vi "Clamp MAX_Setting_UI.vi"(6 "Analysis_Setting IN":T2={"PreProcess"=enum."*Algorithm*", "Parameter"=""}, 8 "error in (no error)":errorcluster, 9 "ProjectName":string, 10 "ROI List IN":refnum<vi>, 11 "Vision_Image":T10(plugin-control)) -> (0 "error out":errorcluster, 1 "Cancel?":bool, 3 "Analysis_Setting":T2={"PreProcess"=enum."*Algorithm*", "Parameter"=""})   [LabVIEW 2019]
uses:
  <vilib>/userdefined/High Color/IMAQdx.ctl
  <vilib>/vision/NI_Vision_Development_Module.lvlib
  Controls/_UI Command Cluster/Clamp MAX_UI Command Cluster.ctl
  Controls/Clamp MAX/Analysis_Clamp MAX_Parameter.ctl
  Controls/Analysis_Type.ctl
  Controls/Analysis_Setting.ctl
  Controls/V_Analysis_Type.ctl
  Ctrl/VisionProcessName.ctl
panel:
  in  "Snap?":bool
  in  "ROI":T1
  in  "Overlay Settings":T4={"Show Search Area"=TRUE, "Show Curves"=TRUE, "Show Clamp Locations"=TRUE, "Show Result"=TRUE, "Search Area Color"=6618880, "Curves Color"=16777224, "Clamp Locations Color"=16776960, "Result Color"=16711680, "Overlay Group Name"=""}
  out "Numeric":i32
  in  "Done":bool
  in  "Clamp MAX_UI Command":T5(ring)
  in  "Cancel":bool
  in  "Clamp MAXTab":T6(tab)
  in  "Clamp Settings":T7={"Angle Range (+/-)"=100.0, "Edge Polarity"={"Start"=0, "End"=0}} {"Edge Polarity"."End" items=["Any", "Rising", "Falling"]; "Edge Polarity"."Start" items=["Any", "Rising", "Falling"]}
  in  "Curve Extraction Settings":T8={"Extraction Mode"=enum."Normal", "Edge Threshold"=40, "Edge Filter Size"=enum."Normal", "Min Length"=15, "Row Search Step Size"=10, "Col Search Step Size"=10, "Max Endpoint Gap"=5, "Closed"=FALSE, "Subpixel"=FALSE} {"Max Endpoint Gap" min=0; "Col Search Step Size" min=1 max=255 step=1; "Row Search Step Size" min=1 max=255 step=1; "Min Length" min=0; "Edge Threshold" min=1 max=350 step=1}
  out "Clamp MAX Results":T9 {"Angle (Relative)" format="%.3f"; "Angle (Absolute)" format="%.3f"; "Distance (Real World)" format="%.3f"; "Distance (Pixels)" format="%.3f"}
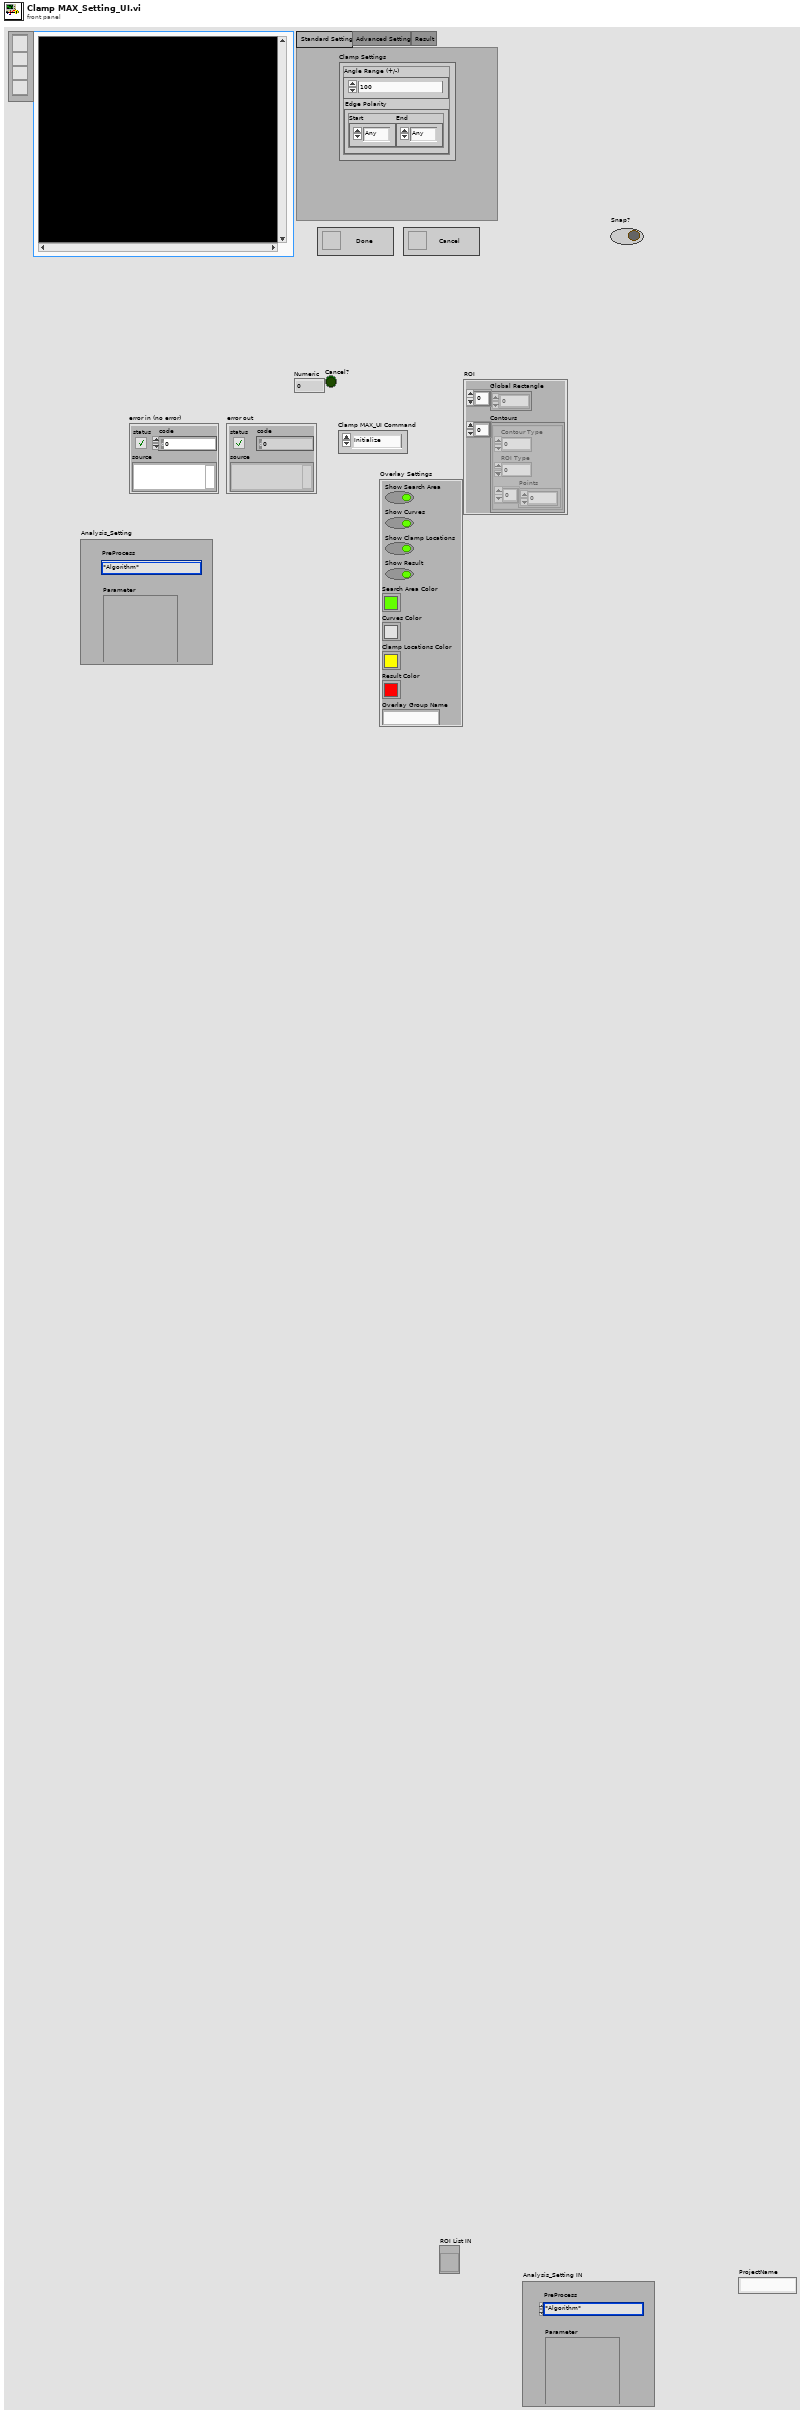
[diagram p1: front panel]
types:
  T1 = cluster{"Global Rectangle":i32[], "Contours":cluster{"Contour Type":u32, "ROI Type":u32, "Points":i32[]}[]}
  T2 = typedef "Analysis_Setting.ctl" = cluster{"PreProcess":T3, "Parameter":string}
  T3 = typedef "VisionProcessName.ctl" = enum16{"*CamParameter*", "CamAttributes", "*Preprocess*", "CG_Brightness", "C_Plane Extraction", "C_Threshold", "G_Lookup Table", "G_Threshold", "B_Image Inversion", "*Algorithm*", "CG_Histogram", "C_Color Matching", "C_Color Pattern Matching", "G_PatternMatch", "CG_Find Straight Edge", "CG_Adv. Find Straight Edge", "CG_Find Circular Edge", "G_Max Clamp", "G_Clamp (Rake)", "G_Pattern Matching"}
  T4 = cluster{"Show Search Area":bool, "Show Curves":bool, "Show Clamp Locations":bool, "Show Result":bool, "Search Area Color":u32, "Curves Color":u32, "Clamp Locations Color":u32, "Result Color":u32, "Overlay Group Name":string}
  T5 = enum16{"Initialize", "Done", "Run Algorithm", "Cancel"}
  T6 = enum32{"Standard Setting", "Advanced Setting", "Result"}
  T7 = cluster{"Angle Range (+/-)":dbl, "Edge Polarity":cluster{"Start":u32, "End":u32}}
  T8 = cluster{"Extraction Mode":enum16{"Normal", "Uniform Regions"}, "Edge Threshold":i32, "Edge Filter Size":enum16{"Fine", "Normal", "Contour Tracing"}, "Min Length":i32, "Row Search Step Size":i32, "Col Search Step Size":i32, "Max Endpoint Gap":i32, "Closed":bool, "Subpixel":bool}
  T9 = cluster{"Distance (Pixels)":dbl, "Distance (Real World)":dbl, "Angle (Absolute)":dbl, "Angle (Relative)":dbl}
  T10 = typedef "IMAQ Image.ctl" = refnum<image>
  T11 = typedef "Clamp MAX_UI Command Cluster.ctl" = cluster{"Clamp MAX_UI Command":enum16{"Initialize", "Done", "Run Algorithm", "Cancel"}, "Overlay Settings":cluster{"Show Search Area":bool, "Show Curves":bool, "Show Clamp Locations":bool, "Show Result":bool, "Search Area Color":u32, "Curves Color":u32, "Clamp Locations Color":u32, "Result Color":u32, "Overlay Group Name":string}, "Curve Extraction Settings":cluster{"Extraction Mode":u32, "Edge Threshold":i32, "Edge Filter Size":u32, "Min Length":i32, "Row Search Step Size":i32, "Col Search Step Size":i32, "Max Endpoint Gap":i32, "Closed":bool, "Subpixel":bool}, "Clamp Settings":cluster{"Angle Range (+/-)":dbl, "Edge Polarity":cluster{"Start":u32, "End":u32}}, "Snap Simulation Mouse Down":bool, "ROI":cluster{"Global Rectangle":i32[], "Contours":cluster{"Contour Type":u32, "ROI Type":u32, "Points":i32[]}[]}}
  T12 = typedef "IMAQ Line" = cluster{"Start X":i32, "Start Y":i32, "End X":i32, "End Y":i32}
  T13 = typedef "IMAQdx.ctl" = refnum<k21>
  T14 = cluster{"Contour Type":u32, "ROI Type":u32, "Points":i32[]}
  T15 = cluster{"Extraction Mode":u32, "Edge Threshold":i32, "Edge Filter Size":u32, "Min Length":i32, "Row Search Step Size":i32, "Col Search Step Size":i32, "Max Endpoint Gap":i32, "Closed":bool, "Subpixel":bool}
  T16 = typedef "Image Type" = u32
  T17 = typedef "Analysis_Clamp MAX_Parameter.ctl" = cluster{"Overlay Settings":cluster{"Show Search Area":bool, "Show Curves":bool, "Show Clamp Locations":bool, "Show Result":bool, "Search Area Color":u32, "Curves Color":u32, "Clamp Locations Color":u32, "Result Color":u32, "Overlay Group Name":string}, "Curve Extraction Settings":cluster{"Extraction Mode":u32, "Edge Threshold":i32, "Edge Filter Size":u32, "Min Length":i32, "Row Search Step Size":i32, "Col Search Step Size":i32, "Max Endpoint Gap":i32, "Closed":bool, "Subpixel":bool}, "Clamp Settings":cluster{"Angle Range (+/-)":dbl, "Edge Polarity":cluster{"Start":u32, "End":u32}}, "ROI":cluster{"Global Rectangle":i32[], "Contours":cluster{"Contour Type":u32, "ROI Type":u32, "Points":i32[]}[]}}
  T18 = typedef "Analysis_Type.ctl" = u16
  T19 = typedef "Analysis_Setting.ctl" = cluster{"PreProcess":T20, "Parameter":string}
  T20 = typedef "V_Analysis_Type.ctl" = enum16{"None", "C_Color Pattern Matching", "G_PatternMatching", "G_ShapeDectect", "G_GeometricMatch", "B_Area Check"}
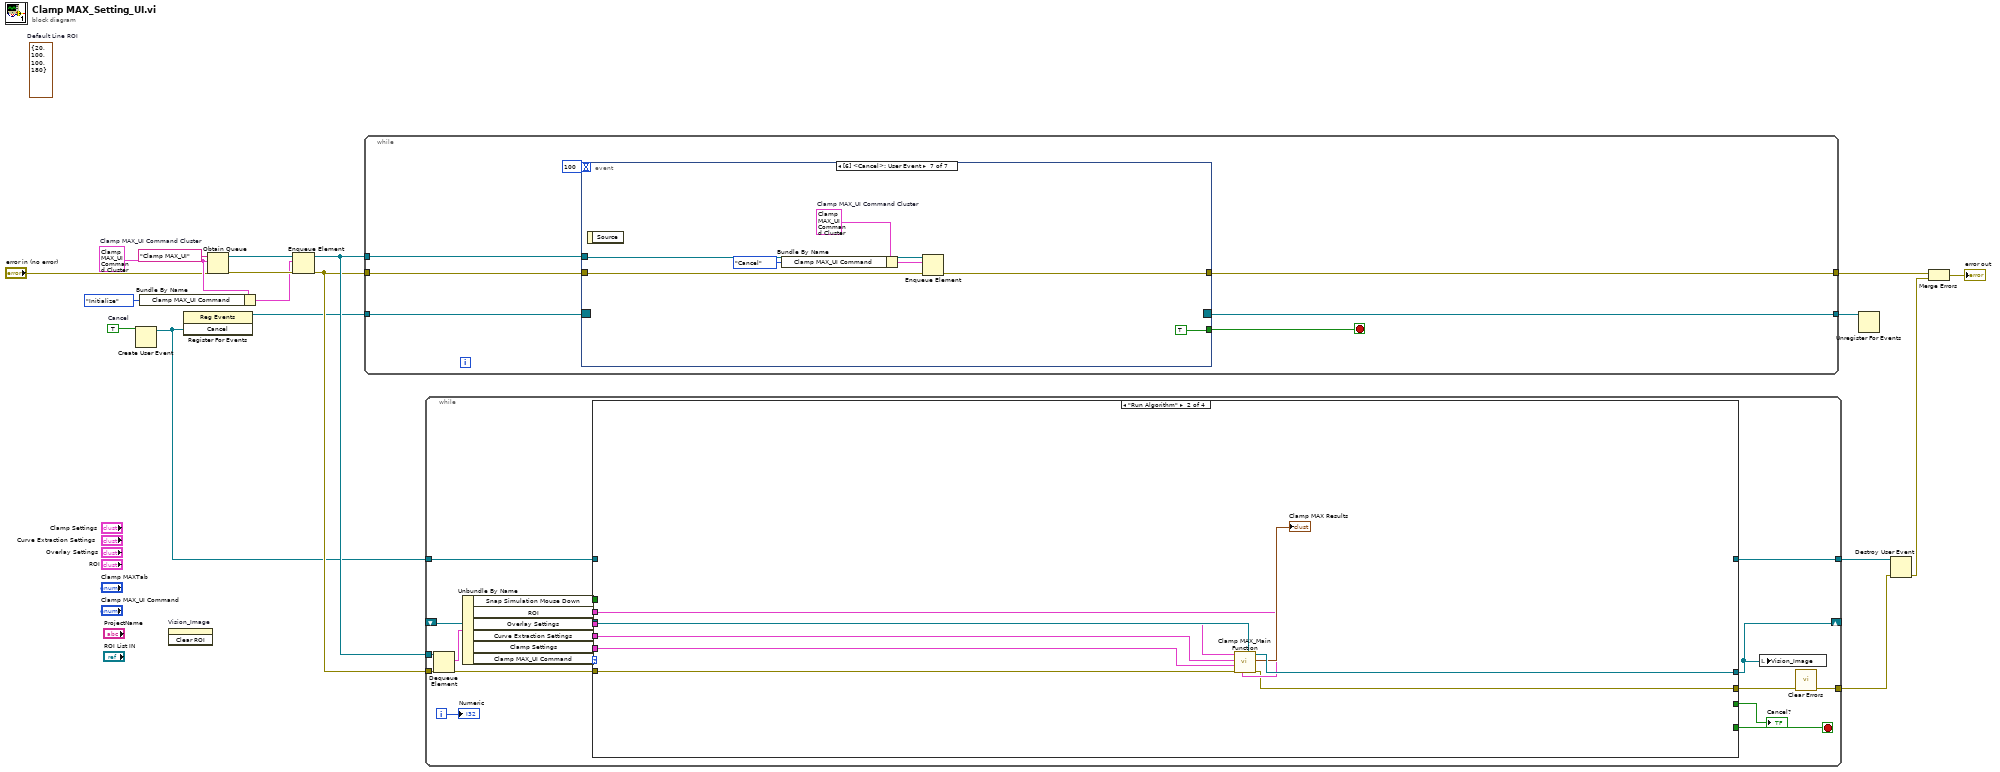
[diagram p0: block diagram]
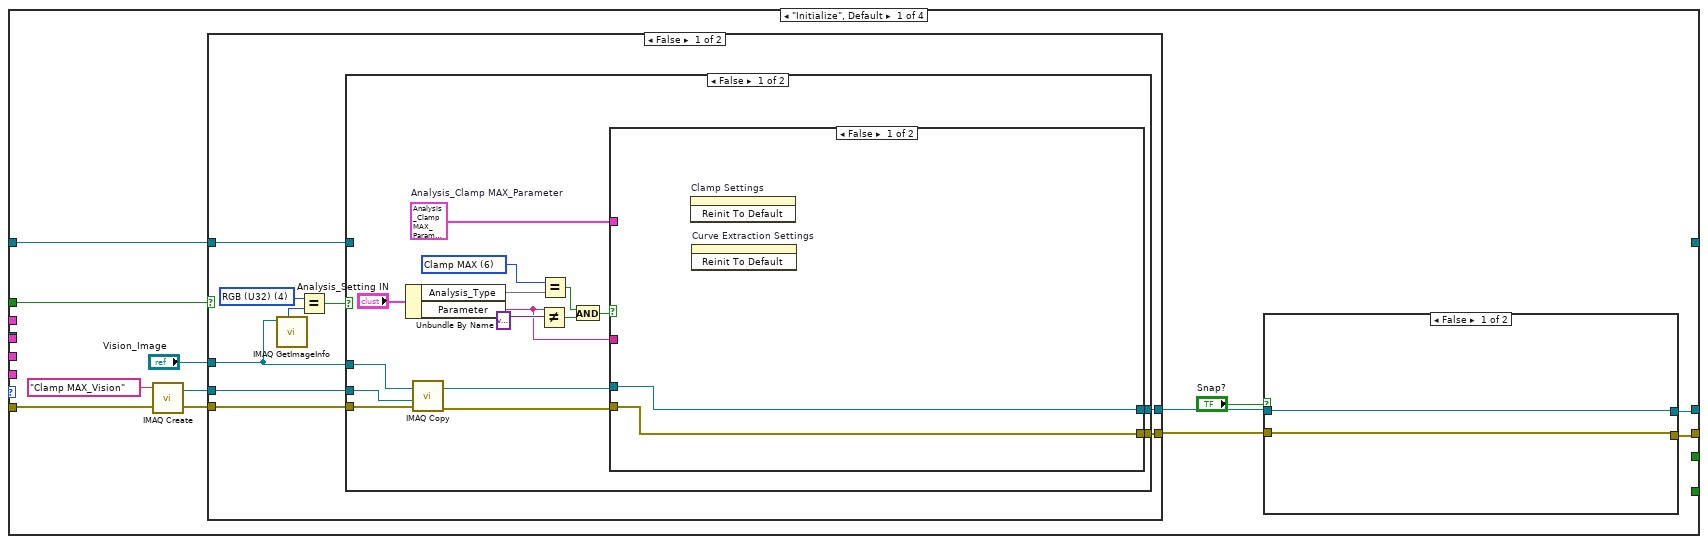
[diagram p2: hidden frame]
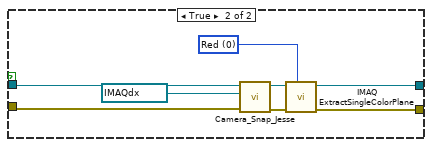
[diagram p3: hidden frame]
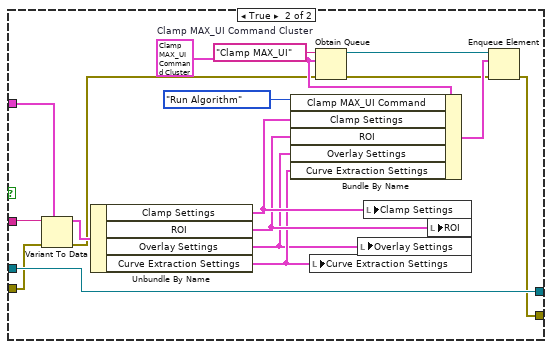
[diagram p4: hidden frame]
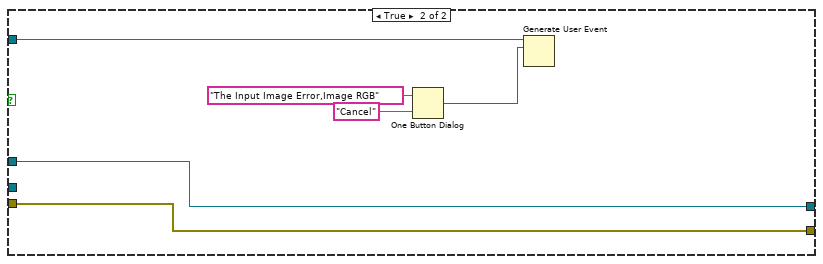
[diagram p5: hidden frame]
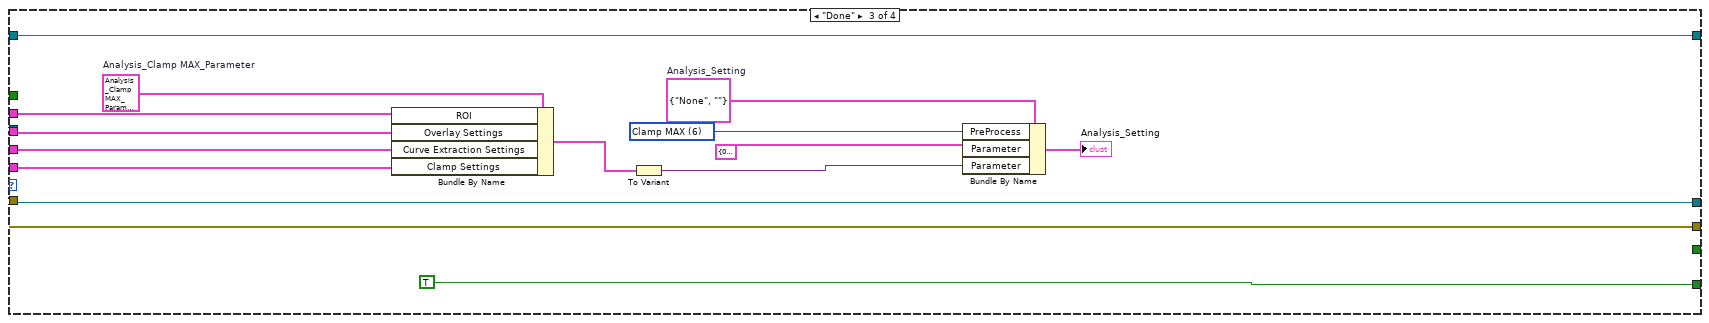
[diagram p7: hidden frame]
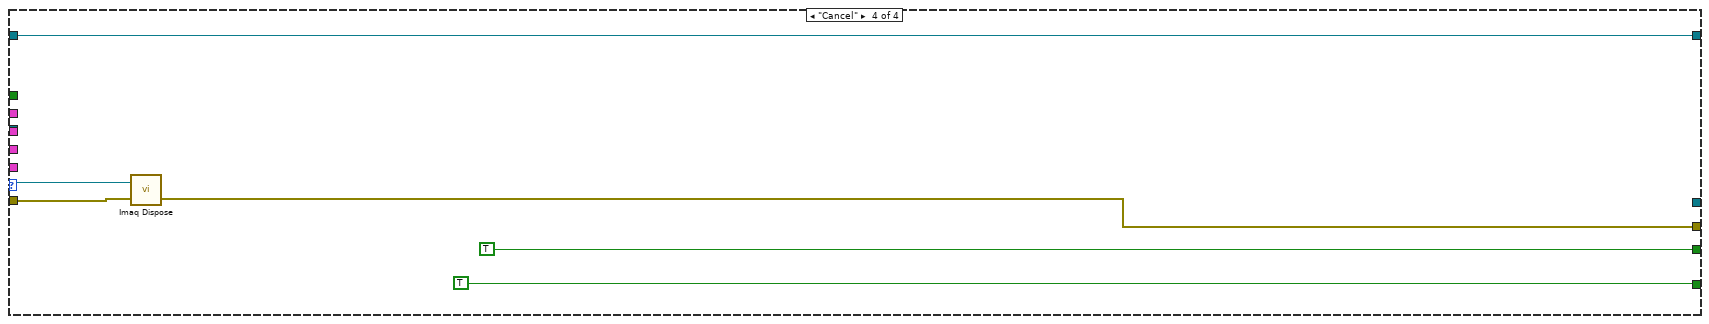
[diagram p8: hidden frame]
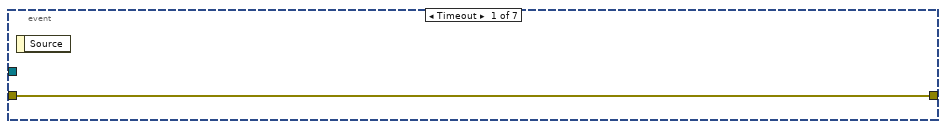
[diagram p9: hidden frame]
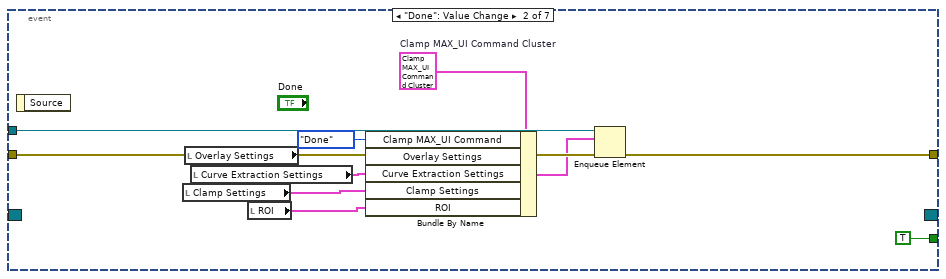
[diagram p10: hidden frame]
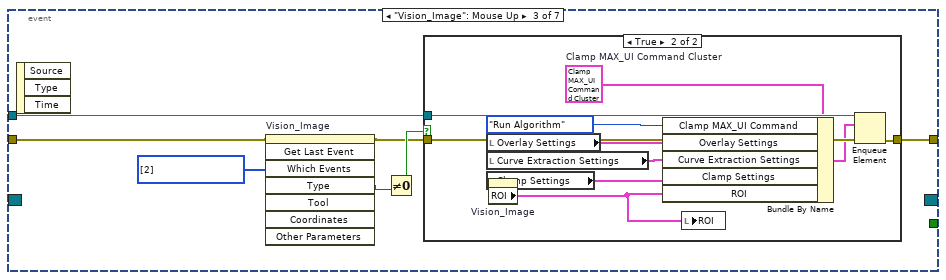
[diagram p11: hidden frame]
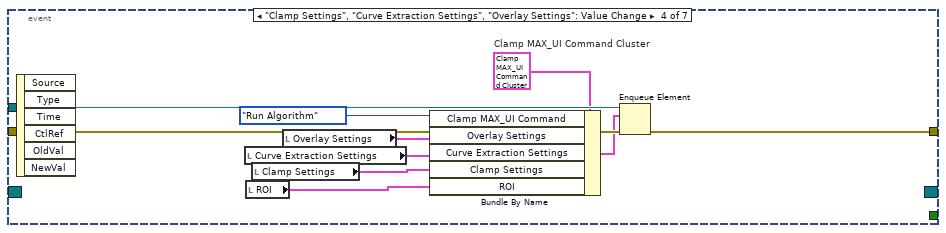
[diagram p13: hidden frame]
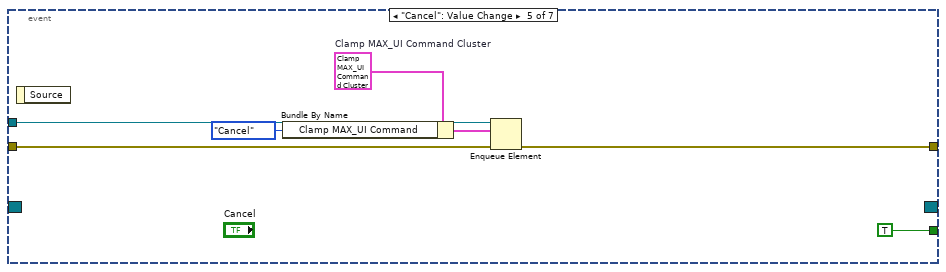
[diagram p14: hidden frame]
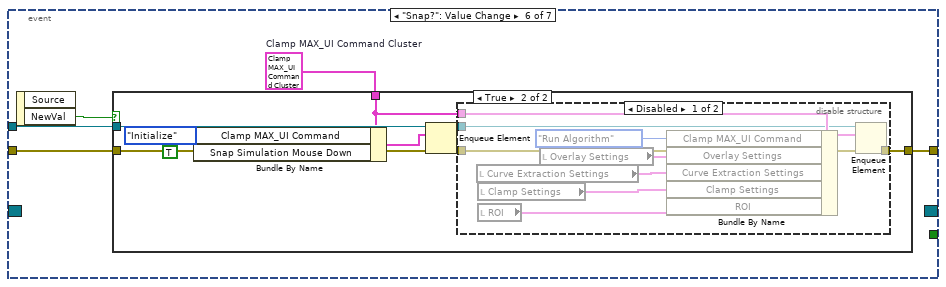
[diagram p15: hidden frame]
diagram:
  w7 = TRUE  # Cancel
  w12 = T11 {"Clamp MAX_UI Command"=enum."Initialize", "Overlay Settings"={"Show Search Area"=TRUE, "Show Curves"=TRUE, "Show Clamp Locations"=TRUE, "Show Result"=TRUE, "Search Area Color"=6618880, "Curves Color"=16777224, "Clamp Locations Color"=16776960, "Result Color"=16711680, "Overlay Group Name"=""}, "Curve Extraction Settings"={"Extraction Mode"=0, "Edge Threshold"=40, "Edge Filter Size"=1, "Min Length"=15, "Row Search Step Size"=10, "Col Search Step Size"=10, "Max Endpoint Gap"=5, "Closed"=FALSE, "Subpixel"=FALSE}, "Clamp Settings"={"Angle Range (+/-)"=5.0, "Edge Polarity"={"Start"=0, "End"=0}}, "Snap Simulation Mouse Down"=FALSE, "ROI"={"Global Rectangle"=[], "Contours"=[]}}  # Clamp MAX_UI Command Cluster
  (unwired) T12 {"Start X"=20, "Start Y"=100, "End X"=100, "End Y"=180}  # Default Line ROI
  n1 = Create User Event(user event datatype=w7) -> (user event=w5:refnum<user-event>)  [unwired: 1 in, 1 out]
  n2 = Bundle By Name(cluster=w12, "Clamp MAX_UI Command"=T5."Initialize" ("Barcode 1D_UI Command")) -> (w13:T11)
  n3 = invoke on="Vision_Image" class="ImageControl" method="Clear ROI"() -> ()  [unwired: 3 in, 3 out]
  n4 = register-events(w5) -> (reference out=w6:refnum<event-registration>)  [unwired: 2 in, 1 out]
  n5 = Obtain Queue(name (unnamed)="Clamp MAX_UI", element data type=w12, error in (no error)="error in (no error)") -> (queue out=w18:refnum<queue>, error out=w17:errorcluster)  [unwired: 2 in, 1 out]
  n6 = Enqueue Element(queue=w18, element=w13, error in (no error)=w17) -> (queue out=w11:refnum<queue>, error out=w10:errorcluster)  [unwired: 1 in, 1 out]
  n7 = while {
    tunnel: w11 -> [w25]
    tunnel: w10 -> [w24]
    tunnel: [w23] -> w15
    tunnel: w6 -> [w20]
    tunnel: [w19] -> w3
    stop <- w21 stop-if-true
    n8 = event shown="[6] <Cancel>: User Event" {
      selector: w20 -> [_ _ _ _ _ _ _]
      dyn-events: [_ _ _ _ _ _ _] -> w19
      timeout: 100 -> [_ _ _ _ _ _ _]
      tunnel: w25 -> [_ w37 w44 w65 w72 w77 w101]
      tunnel: w24 -> [w26 w36 w41 w64 w71 w76 w100]
      tunnel: [_ TRUE _ _ TRUE _ TRUE] -> w21
      tunnel: [w26 w35 w38 w63 w69 w75 w98] -> w23
      event Timeout {
        n9 = event-data() -> ()  [unwired: 1 in, 1 out]
      }
      event "Done": Value Change {
        w34 = T11 {"Clamp MAX_UI Command"=enum."Initialize", "Overlay Settings"={"Show Search Area"=TRUE, "Show Curves"=TRUE, "Show Clamp Locations"=TRUE, "Show Result"=FALSE, "Search Area Color"=6618880, "Curves Color"=16777224, "Clamp Locations Color"=16776960, "Result Color"=16711680, "Overlay Group Name"=""}, "Curve Extraction Settings"={"Extraction Mode"=0, "Edge Threshold"=40, "Edge Filter Size"=1, "Min Length"=15, "Row Search Step Size"=10, "Col Search Step Size"=10, "Max Endpoint Gap"=5, "Closed"=FALSE, "Subpixel"=FALSE}, "Clamp Settings"={"Angle Range (+/-)"=5.0, "Edge Polarity"={"Start"=0, "End"=0}}, "Snap Simulation Mouse Down"=FALSE, "ROI"={"Global Rectangle"=[], "Contours"=[]}}  # Clamp MAX_UI Command Cluster
        n10 = event-data() -> ()  [unwired: 1 in, 1 out]
        n11 = local read "Clamp Settings"() -> (w28:T7)
        n12 = local read "Overlay Settings"() -> (w30:T4)
        n13 = local read "Curve Extraction Settings"() -> (w29:T8)
        n14 = local read "ROI"() -> (w27:T1)
        n15 = Bundle By Name(cluster=w34, "Clamp MAX_UI Command"=T5."Done" ("Edge Detection_UI Command"), "Overlay Settings"=w30, "Curve Extraction Settings"=w29, "Clamp Settings"=w28, "ROI"=w27) -> (w32:T11)
        n16 = Enqueue Element(queue=w37, element=w32, error in (no error)=w36) -> (error out=w35:errorcluster)  [unwired: 1 in, 2 out]
      }
      event "Vision_Image": Mouse Up {
        w42 = i32[] [2] items=["No Event"=0, "Click Event"=1, "Draw Event"=2, "Size Event"=4, "Scroll Event"=5, "Double Click Event"=8] ("Which Events")
        n17 = event-data() -> ()  [unwired: 1 in, 3 out]
        n18 = invoke on="Vision_Image" class="ImageControl" method="Get Last Event"(error in=w41, "Which Events"=w42) -> (error out=w40:errorcluster, "Type"=w39:i32)  [unwired: 6 in, 6 out]
        n19 = Not Equal To 0?(x=w39) -> (x != 0?=w43:bool)
        n20 = case shown="True" w43 {
          tunnel: w44 -> [_ w53]
          tunnel: w40 -> [w45 w55]
          tunnel: [w45 w54] -> w38
          frame False {
          }
          frame True {
            w52 = T11 {"Clamp MAX_UI Command"=enum."Initialize", "Overlay Settings"={"Show Search Area"=TRUE, "Show Curves"=TRUE, "Show Clamp Locations"=TRUE, "Show Result"=TRUE, "Search Area Color"=6618880, "Curves Color"=16777224, "Clamp Locations Color"=16776960, "Result Color"=16711680, "Overlay Group Name"=""}, "Curve Extraction Settings"={"Extraction Mode"=0, "Edge Threshold"=40, "Edge Filter Size"=1, "Min Length"=15, "Row Search Step Size"=10, "Col Search Step Size"=10, "Max Endpoint Gap"=5, "Closed"=FALSE, "Subpixel"=FALSE}, "Clamp Settings"={"Angle Range (+/-)"=5.0, "Edge Polarity"={"Start"=0, "End"=0}}, "Snap Simulation Mouse Down"=FALSE, "ROI"={"Global Rectangle"=[], "Contours"=[]}}  # Clamp MAX_UI Command Cluster
            n21 = local read "Overlay Settings"() -> (w47:T4)
            n22 = local read "Curve Extraction Settings"() -> (w48:T8)
            n23 = local read "Clamp Settings"() -> (w49:T7)
            n24 = property on="Vision_Image" class="ImageControl"() -> ("ROI"=w46:T1)  [unwired: 2 in, 2 out]
            n25 = Bundle By Name(cluster=w52, "Clamp MAX_UI Command"=T5."Run Algorithm", "Overlay Settings"=w47, "Curve Extraction Settings"=w48, "Clamp Settings"=w49, "ROI"=w46) -> (w51:T11)
            n26 = local write "ROI"(w46) -> ()
            n27 = Enqueue Element(queue=w53, element=w51, error in (no error)=w55) -> (error out=w54:errorcluster)  [unwired: 1 in, 2 out]
          }
        }
      }
      event "Clamp Settings", "Curve Extraction Settings", "Overlay Settings": Value Change {
        w62 = T11 {"Clamp MAX_UI Command"=enum."Initialize", "Overlay Settings"={"Show Search Area"=TRUE, "Show Curves"=TRUE, "Show Clamp Locations"=TRUE, "Show Result"=FALSE, "Search Area Color"=6618880, "Curves Color"=16777224, "Clamp Locations Color"=16776960, "Result Color"=16711680, "Overlay Group Name"=""}, "Curve Extraction Settings"={"Extraction Mode"=0, "Edge Threshold"=40, "Edge Filter Size"=1, "Min Length"=15, "Row Search Step Size"=10, "Col Search Step Size"=10, "Max Endpoint Gap"=5, "Closed"=FALSE, "Subpixel"=FALSE}, "Clamp Settings"={"Angle Range (+/-)"=5.0, "Edge Polarity"={"Start"=0, "End"=0}}, "Snap Simulation Mouse Down"=FALSE, "ROI"={"Global Rectangle"=[], "Contours"=[]}}  # Clamp MAX_UI Command Cluster
        n28 = event-data() -> ()  [unwired: 1 in, 6 out]
        n29 = local read "Curve Extraction Settings"() -> (w57:T8)
        n30 = local read "ROI"() -> (w56:T1)
        n31 = local read "Clamp Settings"() -> (w59:T7)
        n32 = local read "Overlay Settings"() -> (w58:T4)
        n33 = Bundle By Name(cluster=w62, "Clamp MAX_UI Command"=T5."Run Algorithm" ("Barcode 1D_UI Command"), "Overlay Settings"=w58, "Curve Extraction Settings"=w57, "Clamp Settings"=w59, "ROI"=w56) -> (w60:T11)
        n34 = Enqueue Element(queue=w65, element=w60, error in (no error)=w64) -> (error out=w63:errorcluster)  [unwired: 1 in, 2 out]
      }
      event "Cancel": Value Change {
        w67 = T11 {"Clamp MAX_UI Command"=enum."Initialize", "Overlay Settings"={"Show Search Area"=TRUE, "Show Curves"=TRUE, "Show Clamp Locations"=TRUE, "Show Result"=FALSE, "Search Area Color"=6618880, "Curves Color"=16777224, "Clamp Locations Color"=16776960, "Result Color"=16711680, "Overlay Group Name"=""}, "Curve Extraction Settings"={"Extraction Mode"=0, "Edge Threshold"=40, "Edge Filter Size"=1, "Min Length"=15, "Row Search Step Size"=10, "Col Search Step Size"=10, "Max Endpoint Gap"=5, "Closed"=FALSE, "Subpixel"=FALSE}, "Clamp Settings"={"Angle Range (+/-)"=5.0, "Edge Polarity"={"Start"=0, "End"=0}}, "Snap Simulation Mouse Down"=FALSE, "ROI"={"Global Rectangle"=[], "Contours"=[]}}  # Clamp MAX_UI Command Cluster
        n35 = event-data() -> ()  [unwired: 1 in, 1 out]
        n36 = Bundle By Name(cluster=w67, "Clamp MAX_UI Command"=T5."Cancel" ("Barcode 1D_UI Command")) -> (w66:T11)
        n37 = Enqueue Element(queue=w72, element=w66, error in (no error)=w71) -> (error out=w69:errorcluster)  [unwired: 1 in, 2 out]
      }
      event "Snap?": Value Change {
        w74 = T11 {"Clamp MAX_UI Command"=enum."Initialize", "Overlay Settings"={"Show Search Area"=TRUE, "Show Curves"=TRUE, "Show Clamp Locations"=TRUE, "Show Result"=FALSE, "Search Area Color"=6618880, "Curves Color"=16777224, "Clamp Locations Color"=16776960, "Result Color"=16711680, "Overlay Group Name"=""}, "Curve Extraction Settings"={"Extraction Mode"=0, "Edge Threshold"=40, "Edge Filter Size"=1, "Min Length"=15, "Row Search Step Size"=10, "Col Search Step Size"=10, "Max Endpoint Gap"=5, "Closed"=FALSE, "Subpixel"=FALSE}, "Clamp Settings"={"Angle Range (+/-)"=5.0, "Edge Polarity"={"Start"=0, "End"=0}}, "Snap Simulation Mouse Down"=FALSE, "ROI"={"Global Rectangle"=[], "Contours"=[]}}  # Clamp MAX_UI Command Cluster
        n38 = event-data() -> ("NewVal"=w73:bool)  [unwired: 1 in, 1 out]
        n39 = case shown="True" w73 {
          tunnel: w77 -> [_ w87]
          tunnel: w76 -> [w78 w86]
          tunnel: w74 -> [_ w84]
          tunnel: [w78 w83] -> w75
          frame False {
          }
          frame True {
            n40 = Bundle By Name(cluster=w84, "Clamp MAX_UI Command"=T5."Initialize" ("Barcode 1D_UI Command"), "Snap Simulation Mouse Down"=TRUE) -> (w82:T11)
            n41 = Enqueue Element(queue=w87, element=w82, error in (no error)=w86) -> (queue out=w80:refnum<queue>, error out=w79:errorcluster)  [unwired: 1 in, 1 out]
            n42 = disable-structure shown="Disabled" {
              disable-tunnel: w84 -> [w97 _]
              disable-tunnel: [w96 _] -> w83
              disable-tunnel: w80 -> [w95 _]
              disable-tunnel: w79 -> [w94 _]
              frame Disabled {
                n43 = local read "Curve Extraction Settings"() -> (w91:T8)
                n44 = local read "Clamp Settings"() -> (w90:T7)
                n45 = local read "ROI"() -> (w88:T1)
                n46 = local read "Overlay Settings"() -> (w92:T4)
                n47 = Bundle By Name(cluster=w97, "Clamp MAX_UI Command"=T5."Run Algorithm" ("Barcode 1D_UI Command"), "Overlay Settings"=w92, "Curve Extraction Settings"=w91, "Clamp Settings"=w90, "ROI"=w88) -> (w89:T11)
                n48 = Enqueue Element(queue=w95, element=w89, error in (no error)=w94) -> (error out=w96:errorcluster)  [unwired: 1 in, 2 out]
              }
              frame Enabled {
              }
            }
          }
        }
      }
      event User Event {
        w103 = T11 {"Clamp MAX_UI Command"=enum."Initialize", "Overlay Settings"={"Show Search Area"=TRUE, "Show Curves"=TRUE, "Show Clamp Locations"=TRUE, "Show Result"=FALSE, "Search Area Color"=6618880, "Curves Color"=16777224, "Clamp Locations Color"=16776960, "Result Color"=16711680, "Overlay Group Name"=""}, "Curve Extraction Settings"={"Extraction Mode"=0, "Edge Threshold"=40, "Edge Filter Size"=1, "Min Length"=15, "Row Search Step Size"=10, "Col Search Step Size"=10, "Max Endpoint Gap"=5, "Closed"=FALSE, "Subpixel"=FALSE}, "Clamp Settings"={"Angle Range (+/-)"=5.0, "Edge Polarity"={"Start"=0, "End"=0}}, "Snap Simulation Mouse Down"=FALSE, "ROI"={"Global Rectangle"=[], "Contours"=[]}}  # Clamp MAX_UI Command Cluster
        n49 = event-data() -> ()  [unwired: 1 in, 1 out]
        n50 = Bundle By Name(cluster=w103, "Clamp MAX_UI Command"=T5."Cancel" ("Barcode 1D_UI Command")) -> (w102:T11)
        n51 = Enqueue Element(queue=w101, element=w102, error in (no error)=w100) -> (error out=w98:errorcluster)  [unwired: 1 in, 2 out]
      }
    }
  }
  n52 = while {
    tunnel: w11 -> [w123]
    tunnel: w10 -> [w122]
    shift-right: [w116] -> _
    shift-left: _ -> [w118]
    tunnel: [w106] -> w2
    tunnel: w5 -> [w108]
    tunnel: [w107] -> w4
    i -> [w117]
    stop <- w109 stop-if-true
    n53 = Dequeue Element(queue=w123, error in (no error)=w122) -> (element=w119:T11, error out=w120:errorcluster)  [unwired: 1 in, 2 out]
    n54 = Unbundle By Name(w119) -> ("Snap Simulation Mouse Down"=w111:bool, "ROI"=w110:T1, "Overlay Settings"=w114:T4, "Curve Extraction Settings"=w113:T15, "Clamp Settings"=w112:T7, "Clamp MAX_UI Command"=w121:T5)
    n55 = case shown="\"Run Algorithm\"" w121 {
      tunnel: w120 -> [w134 w206 w219 w225]
      tunnel: [w125 w198 w219 w224] -> w105
      tunnel: [_ _ TRUE TRUE] -> w109
      tunnel: [w126 w201 w220 _] -> w116
      tunnel: w118 -> [_ w205 w220 w226]
      tunnel: [_ _ _ TRUE] -> w115
      tunnel: w114 -> [_ w204 w217 _]
      tunnel: w113 -> [_ w203 w216 _]
      tunnel: w112 -> [_ w202 w215 _]
      tunnel: w111 -> [w133 _ _ _]
      tunnel: w110 -> [_ w199 w208 _]
      tunnel: w108 -> [w124 _ w207 w222]
      tunnel: [_ _ w207 w222] -> w107
      frame "Initialize", Default {
        n56 = call "IMAQ Create"("Image Name"="Clamp MAX_Vision", "error in (no error)"=w134) -> ("New Image"=w131:T10, "error out"=w132:errorcluster)  [unwired: 3 in]
        n57 = case shown="False" w133 {
          tunnel: [w154 w197] -> w128
          tunnel: [w153 w196] -> w127
          tunnel: w132 -> [w152 w197]
          tunnel: w131 -> [w151 w196]
          tunnel: "Vision_Image" -> [w147 _]
          tunnel: w124 -> [w146 _]
          frame False {
            w149 = T16 4 items=["Grayscale (U8)", "Grayscale (I16)", "Grayscale (SGL)", "Complex (CSG)", "RGB (U32)", "HSL (U32)", "RGB (U64)", "Grayscale (U16)"] ("x")
            n58 = call "IMAQ GetImageInfo"("Image"=w147) -> ("Image Type"=w150:T16)  [unwired: 3 in, 7 out]
            n59 = Equal?(x=w149, y=w150) -> (x = y?=w148:bool)
            n60 = case shown="False" w148 {
              tunnel: [w170 w190] -> w154
              tunnel: [w169 w191] -> w153
              tunnel: w152 -> [w160 w190]
              tunnel: w151 -> [w159 _]
              tunnel: w147 -> [w155 w191]
              tunnel: w146 -> [_ w192]
              frame False {
                w156 = T17 {"Overlay Settings"={"Show Search Area"=FALSE, "Show Curves"=FALSE, "Show Clamp Locations"=FALSE, "Show Result"=FALSE, "Search Area Color"=0, "Curves Color"=0, "Clamp Locations Color"=0, "Result Color"=0, "Overlay Group Name"=""}, "Curve Extraction Settings"={"Extraction Mode"=0, "Edge Threshold"=0, "Edge Filter Size"=0, "Min Length"=0, "Row Search Step Size"=0, "Col Search Step Size"=0, "Max Endpoint Gap"=0, "Closed"=FALSE, "Subpixel"=FALSE}, "Clamp Settings"={"Angle Range (+/-)"=0.0, "Edge Polarity"={"Start"=0, "End"=0}}, "ROI"={"Global Rectangle"=[], "Contours"=[]}}  # Analysis_Clamp MAX_Parameter
                w166 = T18 6 items=["None", "PatternMatch", "Edge Detection", "Barcode 1D", "Barcode 2D", "Clamp", "Clamp MAX", "Particle", "Histogram", "Straight Edge", "Circle", "Shape Detect", "OCR", "Contour", "ColorMatch"] ("x")
                n61 = Unbundle By Name("Analysis_Setting IN") -> ("Analysis_Type"=w165, "Parameter"=w161:string)
                n62 = call "IMAQ Copy"("error in (no error)"=w160, "Image Dst"=w159, "Image Src"=w155) -> ("error out"=w158:errorcluster, "Image Dst Out"=w157:T10)  [unwired: 3 in]
                n63 = Not Equal?(x=w161, y=variant) -> (x != y?=w167:bool)
                n64 = Equal?(x=w166, y=w165) -> (x = y?=w168:bool)
                n65 = And(x=w168, y=w167) -> (x .and. y?=w162:bool)
                n66 = case shown="False" w162 {
                  tunnel: [w171 w173] -> w170
                  tunnel: [w172 w189] -> w169
                  tunnel: w158 -> [w171 w175]
                  tunnel: w157 -> [w172 w189]
                  tunnel: w161 -> [_ w188]
                  tunnel: w156 -> [_ w178]
                  frame False {
                    n67 = invoke on="Clamp Settings" class="Clust (strict)" method="Reinit To Default"() -> ()  [unwired: 3 in, 3 out]
                    n68 = invoke on="Curve Extraction Settings" class="Clust (strict)" method="Reinit To Default"() -> ()  [unwired: 3 in, 3 out]
                  }
                  frame True {
                    w186 = T11 {"Clamp MAX_UI Command"=enum."Initialize", "Overlay Settings"={"Show Search Area"=TRUE, "Show Curves"=TRUE, "Show Clamp Locations"=TRUE, "Show Result"=TRUE, "Search Area Color"=6618880, "Curves Color"=16777224, "Clamp Locations Color"=16776960, "Result Color"=16711680, "Overlay Group Name"=""}, "Curve Extraction Settings"={"Extraction Mode"=0, "Edge Threshold"=40, "Edge Filter Size"=1, "Min Length"=15, "Row Search Step Size"=10, "Col Search Step Size"=10, "Max Endpoint Gap"=5, "Closed"=FALSE, "Subpixel"=FALSE}, "Clamp Settings"={"Angle Range (+/-)"=5.0, "Edge Polarity"={"Start"=0, "End"=0}}, "Snap Simulation Mouse Down"=FALSE, "ROI"={"Global Rectangle"=[], "Contours"=[]}}  # Clamp MAX_UI Command Cluster
                    n69 = Variant To Data(error in=w175, type=w178, Variant=w188) -> (data=w187:T17, error out=w174:errorcluster)
                    n70 = Unbundle By Name(w187) -> ("Clamp Settings"=w180:T7, "ROI"=w179:T1, "Overlay Settings"=w176:T4, "Curve Extraction Settings"=w177:T15)
                    n71 = Bundle By Name(cluster=w186, "Clamp MAX_UI Command"=T5."Run Algorithm" ("Barcode 1D_UI Command"), "Clamp Settings"=w180, "ROI"=w179, "Overlay Settings"=w176, "Curve Extraction Settings"=w177) -> (w185:T11)
                    n72 = local write "Curve Extraction Settings"(w177) -> ()
                    n73 = Obtain Queue(name (unnamed)="Clamp MAX_UI", element data type=w186, error in (no error)=w174) -> (queue out=w181:refnum<queue>, error out=w182:errorcluster)  [unwired: 2 in, 1 out]
                    n74 = local write "Overlay Settings"(w176) -> ()
                    n75 = local write "Clamp Settings"(w180) -> ()
                    n76 = local write "ROI"(w179) -> ()
                    n77 = Enqueue Element(queue=w181, element=w185, error in (no error)=w182) -> (error out=w173:errorcluster)  [unwired: 1 in, 2 out]
                  }
                }
              }
              frame True {
                n78 = One Button Dialog(message="The Input Image Error,Image RGB", button name ("OK")="Cancel") -> (true=w193:bool)
                n79 = Generate User Event(user event=w192, event data cluster=w193) -> ()  [unwired: 2 in, 2 out]
              }
            }
          }
          frame True {
          }
        }
        n80 = case shown="False" "Snap?" {
          tunnel: [w136 w141] -> w125
          tunnel: [w137 w140] -> w126
          tunnel: w128 -> [w136 w138]
          tunnel: w127 -> [w137 w139]
          frame False {
          }
          frame True {
            w143 = 0 items=["Red", "Green", "Blue", "Hue", "Saturation", "Luminance", "Value", "Intensity"] ("Color Plane")
            n81 = call "Camera_Snap_Jesse.vi"("error in (no error)"=w138, "Camera Session In"=T13 "cam01", "Image In"=w139) -> ("error out"=w142:errorcluster, "New Image"=w144:T10)  [unwired: 7 in]
            n82 = call "IMAQ ExtractSingleColorPlane"("Color Plane"=w143, "error in (no error)"=w142, "Image Src"=w144) -> ("error out"=w141:errorcluster, "Image Dst Out"=w140:T10)  [unwired: 1 in, 6 out]
          }
        }
      }
      frame "Run Algorithm" {
        n83 = call "Clamp MAX_Main Function.vi"("Refnum in"=w205, "ROI"=w199, "error in (no error)"=w206, "Clamp Settings in"=w202, "Curve Extraction Settings in"=w203, "Overlay Settings"=w204) -> ("error out"=w198:errorcluster, "Clamp Results"=→"Clamp MAX Results":T9, "Refnum out"=w201:T10)  [unwired: 2 in, 1 out]
      }
      frame "Done" {
        w209 = T18 6 items=["None", "PatternMatch", "Edge Detection", "Barcode 1D", "Barcode 2D", "Clamp", "Clamp MAX", "Particle", "Histogram", "Straight Edge", "Circle", "Shape Detect", "OCR", "Contour", "ColorMatch"] ("Analysis_Type")
        w214 = T19 {"PreProcess"=enum."None", "Parameter"=""}  # Analysis_Setting
        w218 = T17 {"Overlay Settings"={"Show Search Area"=TRUE, "Show Curves"=TRUE, "Show Clamp Locations"=TRUE, "Show Result"=TRUE, "Search Area Color"=5, "Curves Color"=2, "Clamp Locations Color"=0, "Result Color"=0, "Overlay Group Name"=""}, "Curve Extraction Settings"={"Extraction Mode"=0, "Edge Threshold"=0, "Edge Filter Size"=0, "Min Length"=0, "Row Search Step Size"=0, "Col Search Step Size"=0, "Max Endpoint Gap"=0, "Closed"=FALSE, "Subpixel"=FALSE}, "Clamp Settings"={"Angle Range (+/-)"=40.0, "Edge Polarity"={"Start"=0, "End"=0}}, "ROI"={"Global Rectangle"=[], "Contours"=[]}}  # Analysis_Clamp MAX_Parameter
        n84 = Bundle By Name(cluster=w218, "ROI"=w208, "Overlay Settings"=w217, "Curve Extraction Settings"=w216, "Clamp Settings"=w215) -> (w212:T17)
        n85 = To Variant(anything=w212) -> (Variant=w211:variant)
        n86 = Bundle By Name(cluster=w214, "PreProcess"=w209, "Parameter"=T14 {"Contour Type"=0, "ROI Type"=0, "Points"=[]} ("RegionContour"), "Parameter"=w211) -> (→"Analysis_Setting":T19)
      }
      frame "Cancel" {
        n87 = call "Imaq Dispose"("Image"=w226, "error in (no error)"=w225) -> ("error out"=w224:errorcluster)  [unwired: 4 in]
      }
    }
    "Cancel?" <- w115
    n88 = local write "Vision_Image"(w116) -> ()
    n89 = call <vilib>:"Clear Errors.vi"("error in (no error)"=w105) -> ("error out"=w106:errorcluster)  [unwired: 5 in, 1 out]
    "Numeric" <- w117
  }
  n90 = Unregister For Events(event registration refnum=w3) -> ()  [unwired: 1 in, 1 out]
  n91 = Destroy User Event(user event=w4, error in=w2) -> (error out=w1:errorcluster)
  n92 = Merge Errors(w15, w1) -> (→"error out":errorcluster)
